vi "Is U8 changed.vi"(3 "in":u8) -> (1 "changed or first call?":bool)   [LabVIEW 2019, in "Logik.lvlib"]
uses:
  Logik.lvlib
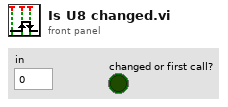
[diagram p1: front panel]
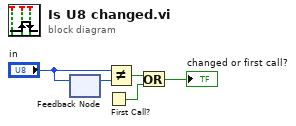
[diagram p0: block diagram]
diagram:
  n1 = feedback-in #1("in") -> ()
  n2 = feedback #1() -> (w5:u8)  [unwired: 1 in]
  n3 = First Call?() -> (First Call?: T/F=w2:bool)
  n4 = Not Equal?(x="in", y=w5) -> (x != y?=w3:bool)
  n5 = Or(x=w3, y=w2) -> (x .or. y?=→"changed or first call?":bool)
